vi "Assert.vi"(6 "error code (1)":i32=1, 7 "Name":string, 8 "error in (no error)":errorcluster, 10 "Assert?":bool, 11 "Assert in":refnum<class "Test Assert.lvclass">) -> (0 "error out":errorcluster, 3 "Assert out":refnum<class "Test Assert.lvclass">)   [LabVIEW 2009, in "Caraya.lvlib" / "Test Assert.lvclass"]
doc: "Assertion implenetation for unit testing. Publishes results of assertion to the unit test framework."
uses:
  Test Assert.lvclass
  Assert/Assert.lvclass
  Assert Factory/Assert Factory.lvclass
  Test Manager/Test Manager.lvclass
  Assert Factory Global/Assert Factory Global.lvclass
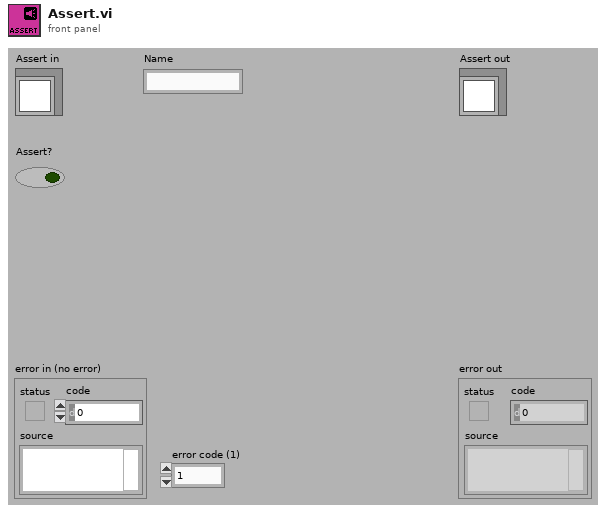
[diagram p1: front panel]
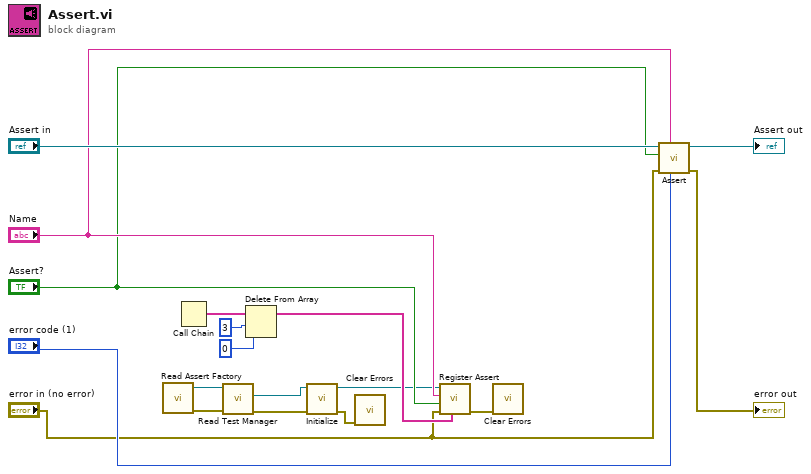
[diagram p0: block diagram]
diagram:
  n1 = call "Read Assert Factory.vi"() -> ("error out"=w12:errorcluster, "Assert Factory"=w11:refnum<class "Assert Factory.lvclass">)  [unwired: 10 in]
  n2 = Call Chain() -> (call chain=w10:string[])
  n3 = call-dynamic "Read Test Manager.vi"("error in (no error)"=w12, "Assert Factory in"=w11) -> ("error out"=w6:errorcluster, "Test Manager"=w4:refnum<class "Test Manager.lvclass">)  [unwired: 7 in, 1 out]
  n4 = Delete From Array(array=w10, length=3 ("index"), index=0) -> (array with subset deleted=w9:string[])  [unwired: 1 out]
  n5 = call-dynamic "Initialize.vi"("error in (no error)"=w6, "Test Manager in"=w4) -> ("error out"=w3:errorcluster, "Test Manager out"=w5:refnum<class "Test Manager.lvclass">)  [unwired: 8 in]
  n6 = call <vilib>:"Clear Errors.vi"("error in (no error)"=w3) -> ()  [unwired: 6 in, 1 out]
  n7 = call-dynamic "Register Assert.vi"("Call Chain"=w9, "error in (no error)"="error in (no error)", "Succeeded"="Assert?", "Message"="Name", "Test Manager in"=w5) -> ("error out"=w1:errorcluster)  [unwired: 5 in, 1 out]
  n8 = call <vilib>:"Clear Errors.vi"("error in (no error)"=w1) -> ()  [unwired: 6 in, 1 out]
  n9 = call-parent "Assert.vi"("error code (1)"="error code (1)", "Name"="Name", "error in (no error)"="error in (no error)", "Assert?"="Assert?", "Assert in"="Assert in") -> ("error out"=→"error out":errorcluster, "Assert out"=→"Assert out":refnum<class "Test Assert.lvclass">)  [unwired: 5 in]
